vi "temp chart calculations.vi"(0 "temp in":dbl format="%.2f", 7 "Control Parameters":T1={"Setpoint"=50.0, "Control bandwidth"=4.0, "Settle bandwidth"=1.0} {"Settle bandwidth" format="%.2f"; "Control bandwidth" format="%.2f"; "Setpoint" format="%.2f"}, 9 "Temperature History in":refnum<vi>, 11 "norm power in":dbl format="%.2f", 13 "Mode":enum16{"Expanded", "Shrunk"}(ring)) -> (4 "Temperature History":T3 {"?" format="%.2f"; "?" format="%.2f"; "?" format="%.2f"; "?" format="%.2f"; "?" format="%.2f"; "?" format="%.2f"; "temp out" format="%.2f"}, 8 "range indicators":T2={"In control band"=TRUE, "In settle band"=TRUE, "under range"=TRUE, "over range"=TRUE}, 10 "Temperature History out":refnum<vi>)   [LabVIEW 2014]
doc: "This subvi does various calculations for the temperature controller display\n\nMatt Strader\nPaul K Dixon\nPhysics 350\nPaul K Dixon"
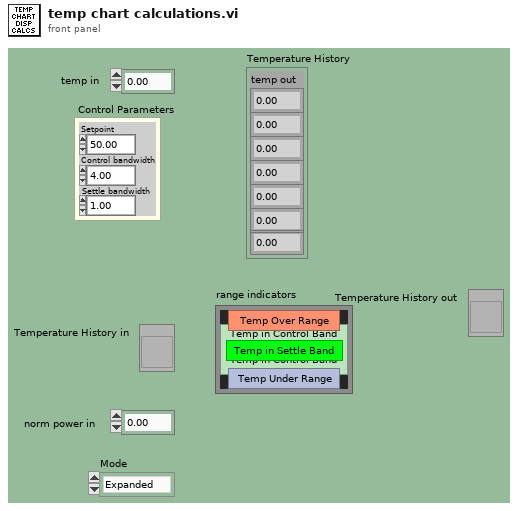
[diagram p1: front panel]
types:
  T1 = cluster{"Setpoint":dbl, "Control bandwidth":dbl, "Settle bandwidth":dbl}
  T2 = cluster{"In control band":bool, "In settle band":bool, "under range":bool, "over range":bool}
  T3 = cluster{"temp out":dbl, dbl, dbl, dbl, dbl, dbl, dbl}
  T4 = cluster{"temp in":dbl, "Setpoint":dbl, "THC":dbl, "TLC":dbl, "THS":dbl, "TLS":dbl, dbl}
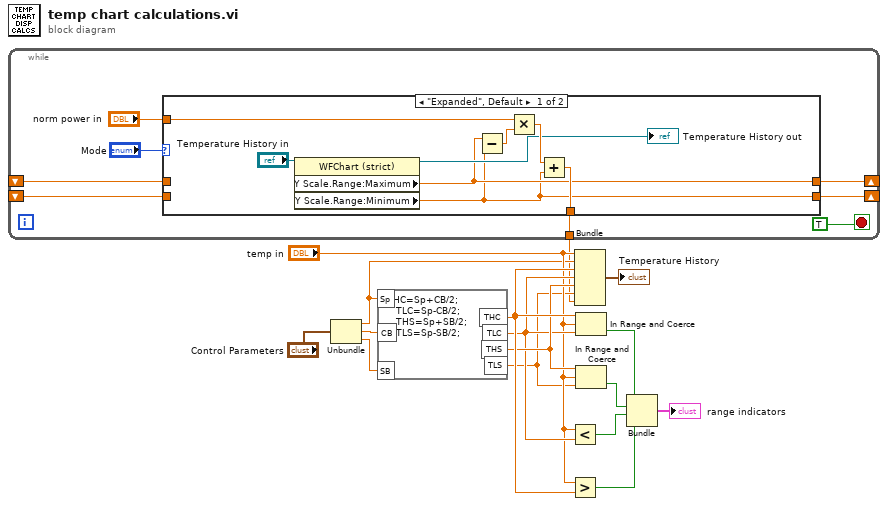
[diagram p0: block diagram]
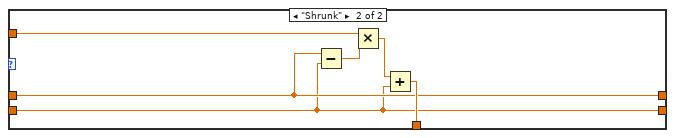
[diagram p2: hidden frame]
diagram:
  n1 = while {
    tunnel: [w24] -> w7
    shift-right: [w20] -> _
    shift-left: _ -> [w18]
    shift-right: [w19] -> _
    shift-left: _ -> [w17]
    stop <- TRUE stop-if-true
    n2 = case shown="\"Expanded\", Default" "Mode" {
      tunnel: [w31 w37] -> w24
      tunnel: "norm power in" -> [w27 w35]
      tunnel: [w26 w34] -> w20
      tunnel: [w25 w33] -> w19
      tunnel: w18 -> [_ w34]
      tunnel: w17 -> [_ w33]
      frame "Expanded", Default {
        n3 = property class="WFChart (strict)"(reference="Temperature History in") -> (reference out=→"Temperature History out":refnum<vi>, "Y Scale.Range:Maximum"=w26:dbl, "Y Scale.Range:Minimum"=w25:dbl)  [unwired: 1 in, 1 out]
        n4 = Subtract(x=w26, y=w25) -> (x-y=w30:dbl)
        n5 = Multiply(x=w27, y=w30) -> (x*y=w32:dbl)
        n6 = Add(x=w32, y=w25) -> (x+y=w31:dbl)
      }
      frame "Shrunk" {
        n7 = Subtract(x=w34, y=w33) -> (x-y=w36:dbl)
        n8 = Multiply(x=w35, y=w36) -> (x*y=w38:dbl)
        n9 = Add(x=w38, y=w33) -> (x+y=w37:dbl)
      }
    }
  }
  n10 = Unbundle("Control Parameters") -> ("Setpoint"=w11:dbl, "Control bandwidth"=w9:dbl, "Settle bandwidth"=w10:dbl)
  n11 = formula code="THC=Sp+CB/2;\n   TLC=Sp-CB/2;\n   THS=Sp+SB/2;\n   TLS=Sp-SB/2;"("Sp"=w11, "CB"=w9, "SB"=w10) -> ("THC"=w16:dbl, "TLC"=w14:dbl, "THS"=w15:dbl, "TLS"=w8:dbl)
  n12 = Less?(x="temp in", y=w14) -> (x < y?=w4:bool)
  n13 = Greater?(x="temp in", y=w16) -> (0:w5:bool)
  n14 = Bundle("temp in"="temp in", "Setpoint"=w11, "THC"=w16, "TLC"=w14, "THS"=w15, "TLS"=w8, w7) -> (→"Temperature History":T4)  [unwired: 1 out]
  n15 = In Range and Coerce(upper limit=w16, x="temp in", lower limit=w14) -> (In Range?=w6:bool)  [unwired: 1 out]
  n16 = In Range and Coerce(upper limit=w15, x="temp in", lower limit=w8) -> (In Range?=w3:bool)  [unwired: 1 out]
  n17 = Bundle(w6, w3, w4, w5) -> (→"range indicators":cluster{bool, bool, bool, bool})  [unwired: 1 out]
